vi "Main.vi"() -> ()   [LabVIEW 2013]
doc: "Use this template to build a simple state machine design pattern. Each state executes code and determines which state to transition to."
uses:
  <vilib>/express/express shared/transition.llb/Dynamic To Waveform Array.vi
  <vilib>/express/express shared/transition.llb/Waveform Array To Dynamic.vi
  <vilib>/express/express arith-compare/Formula/Block/exnFormulaBlock how many pts in the wave.vi
  <vilib>/express/express shared/ex_Modify Signal Name.vi
  <vilib>/express/express arith-compare/Formula/XNode/ExpressFormulaBlockNode.xnode
panel:
  out "Pwm Chart":i16(graph)
  out "PWM On":bool
  out "Mass Flow":dbl
  out "Bare, Coated, and DC":T1(graph)
  out "RecCount":i32
  in  "Period (ms)":dbl=3.0
  out "Coated Temperature":dbl
  out "Bare Temperature":dbl
  out "Low Airflow":bool
  in  "Stop":bool=TRUE
  in  "Filename to save to":path=path "Z:/adit/Desktop/MEL III/RefrigerationData.lvm" caption="Filename"
  in  "Save Data?":bool=TRUE
  out "Derivative Output":dbl
  out "Integral Output":dbl
  out "CO Bias":dbl
  out "Proportional Output":dbl
  out "Duty Cycle":dbl
  out "Current Set Point":dbl
  in  "Integral Constant":dbl=0.1 caption="I Coefficient" format="%0.2f"
  in  "Derivative \nConstant":dbl=0.05 caption="D Coefficient" format="%0.2f"
  in  "Proportional\nConstant":dbl=1.0 caption="P Coefficient" format="%0.2f"
  in  "Duty Cycle\nincrement amount":dbl=1.0
  in  "Decrease Duty Cycle":bool
  in  "Increase Duty Cycle":bool
  in  "Set Point\nIncrement amount":dbl=1.0
  in  "Lower Set Point":bool
  in  "Raise Set Point":bool
  in  "Bare(T) or \nCoated?":bool
  in  "Manual / Auto":bool
  in  "Time to wait(ms)":u32
  in  "Readings between\nrecorded data":i32
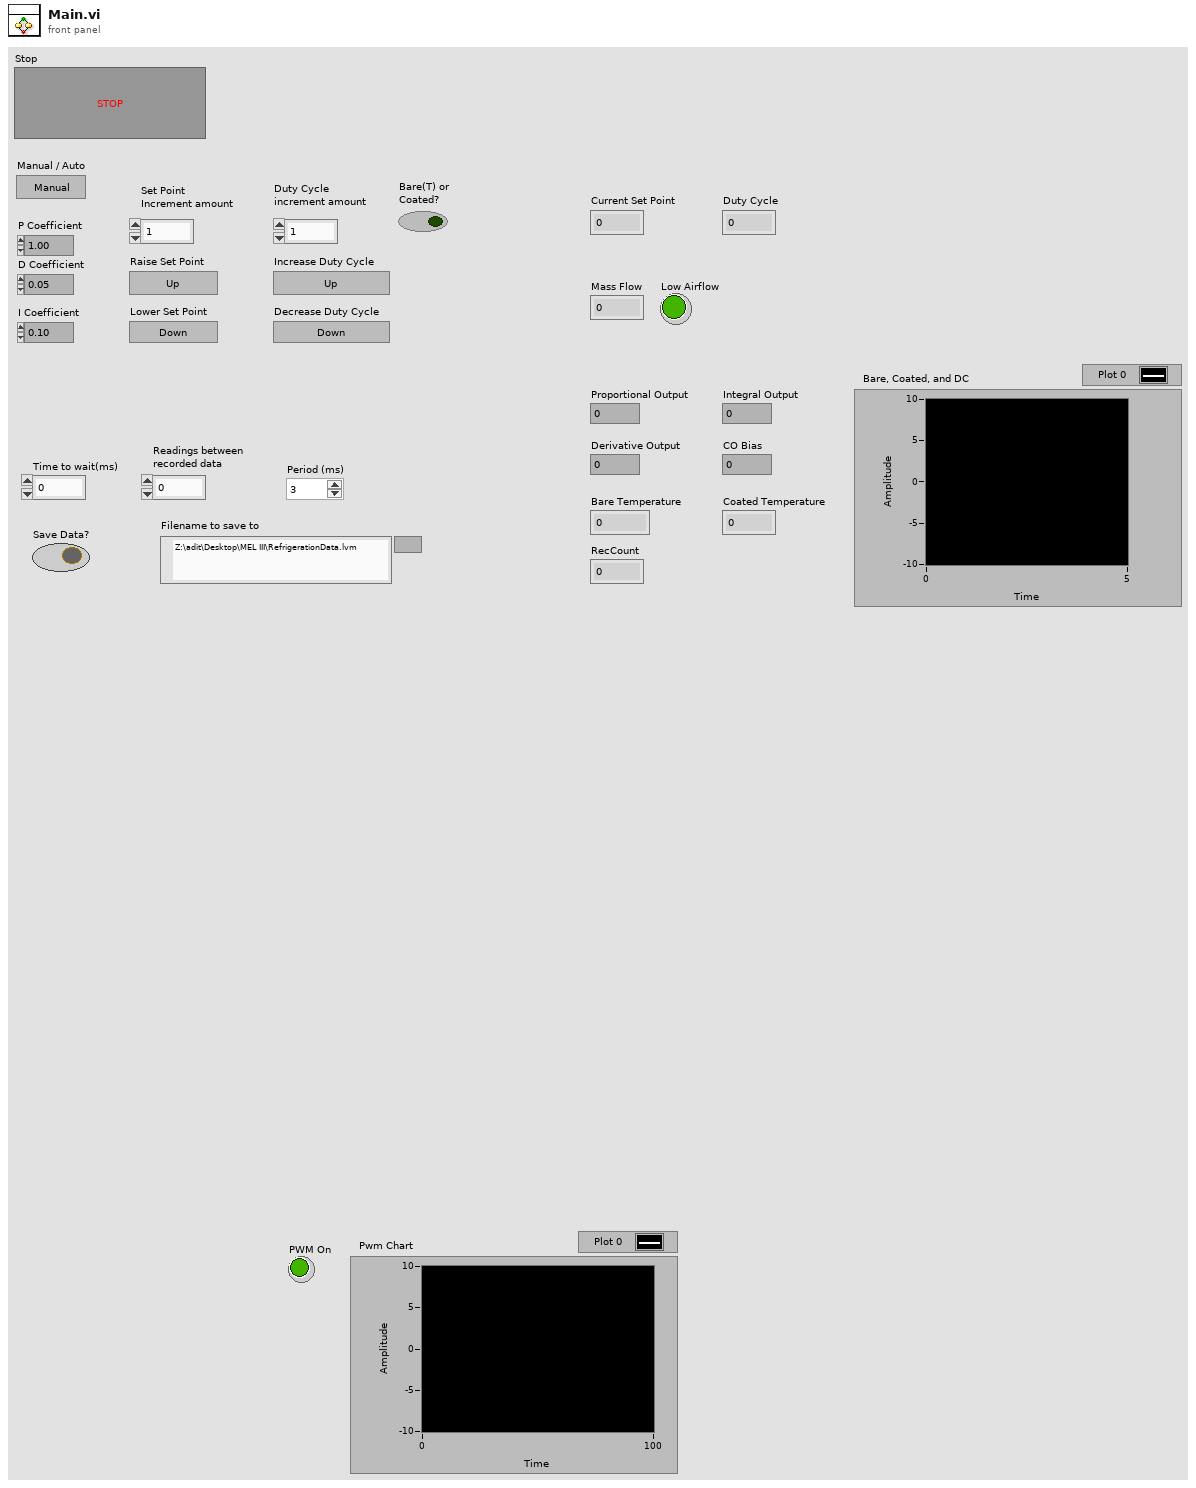
[diagram p1: front panel]
types:
  T1 = cluster{"Uncoated Probe":dbl, "Coated Probe":dbl, "Duty Cycle":dbl}
  T2 = cluster{"RecCount":i32, "Starting Tick Count":i32, "Coated Probe":dbl, "Uncoated Probe":dbl, "Mass Flow":dbl, "Derivative Out":dbl, "Integral Out":dbl, "Proportional Out":dbl, "Manual/Auto":bool, "Set Point":dbl, "Duty Cycle":dbl, "Pwm Value":bool}
  T3 = enum16{"Initialize", "Acquire", "Analyze", "PID", "Record", "PWM", "Output", ""}
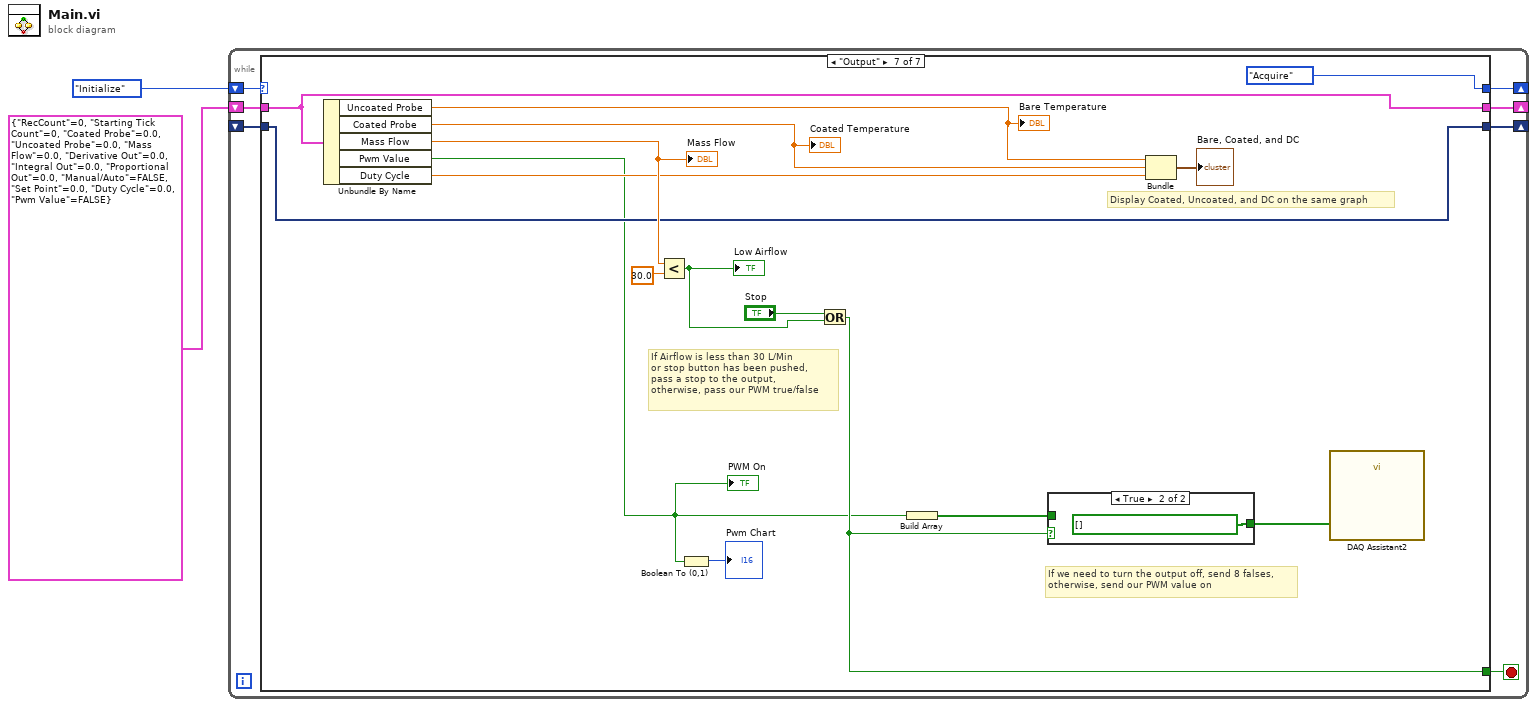
[diagram p0: block diagram]
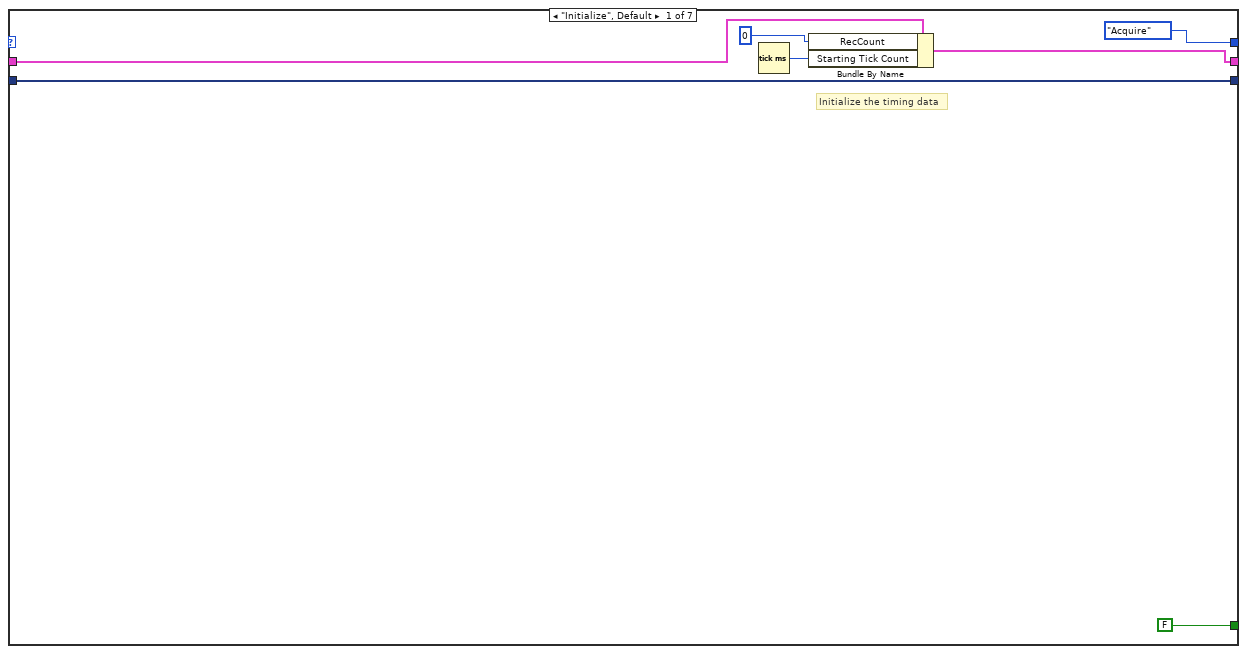
[diagram p2: hidden frame]
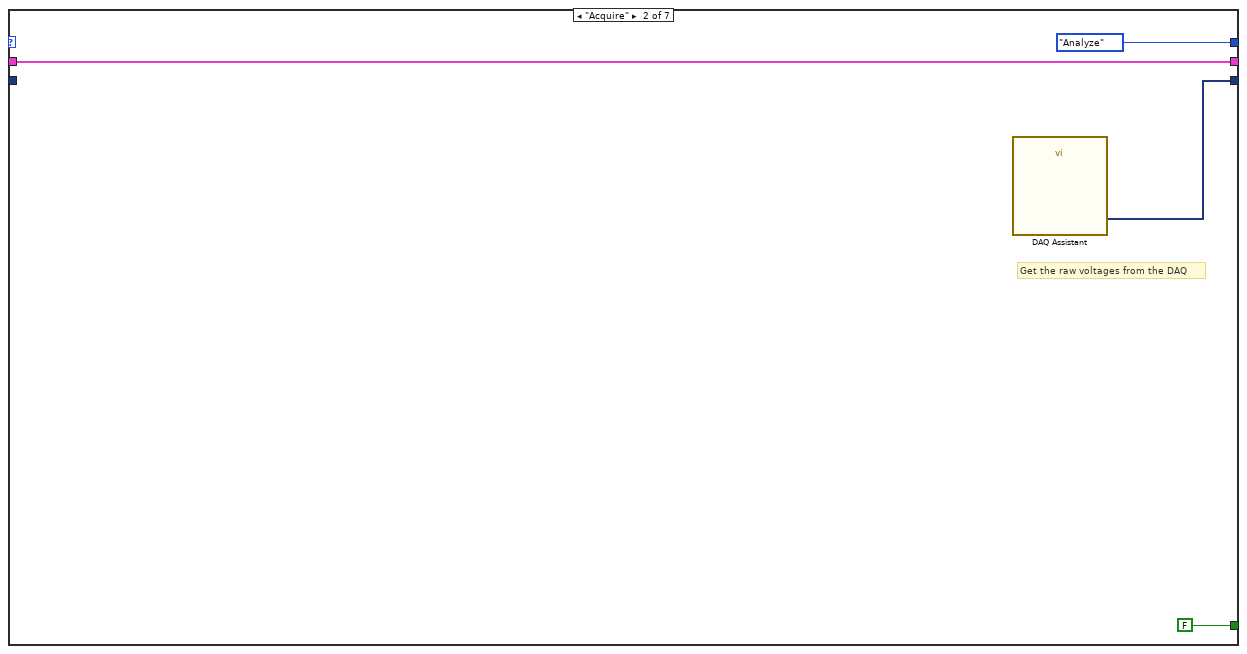
[diagram p3: hidden frame]
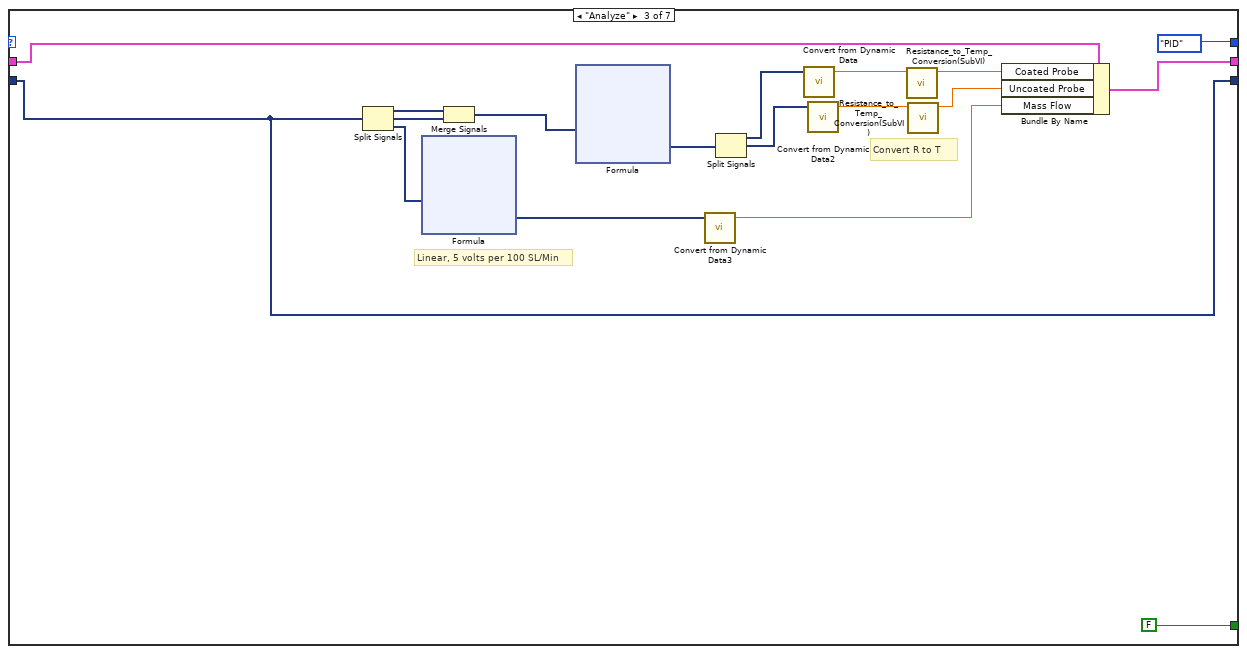
[diagram p4: hidden frame]
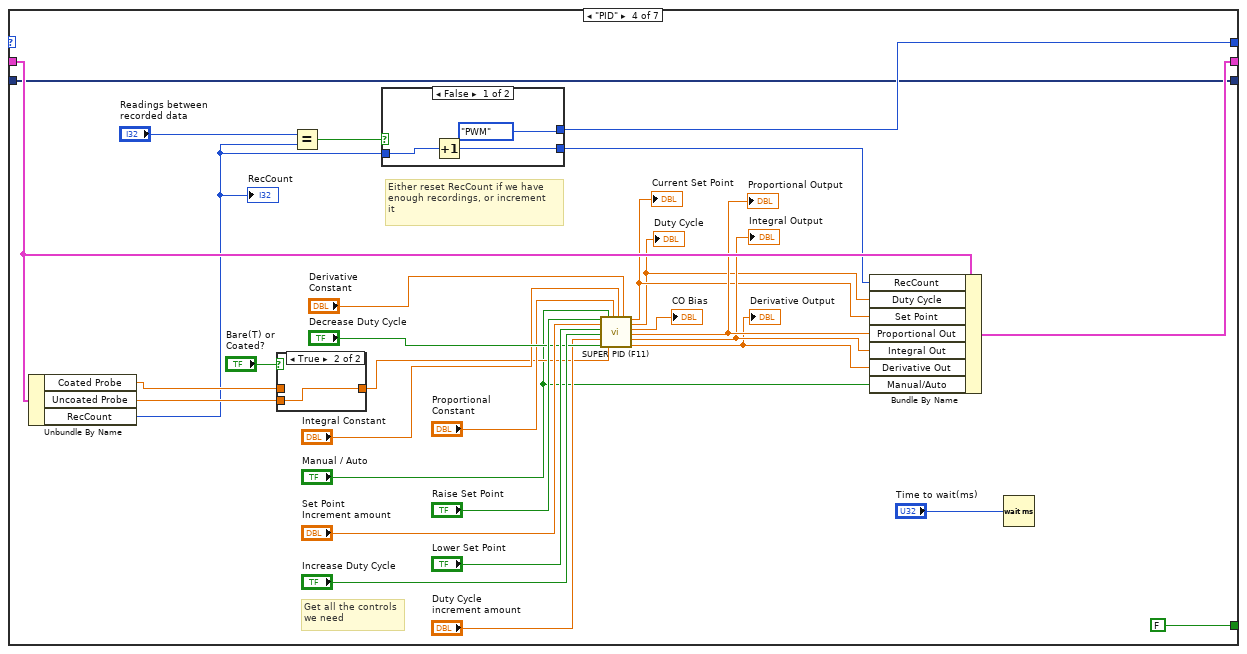
[diagram p5: hidden frame]
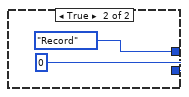
[diagram p7: hidden frame]
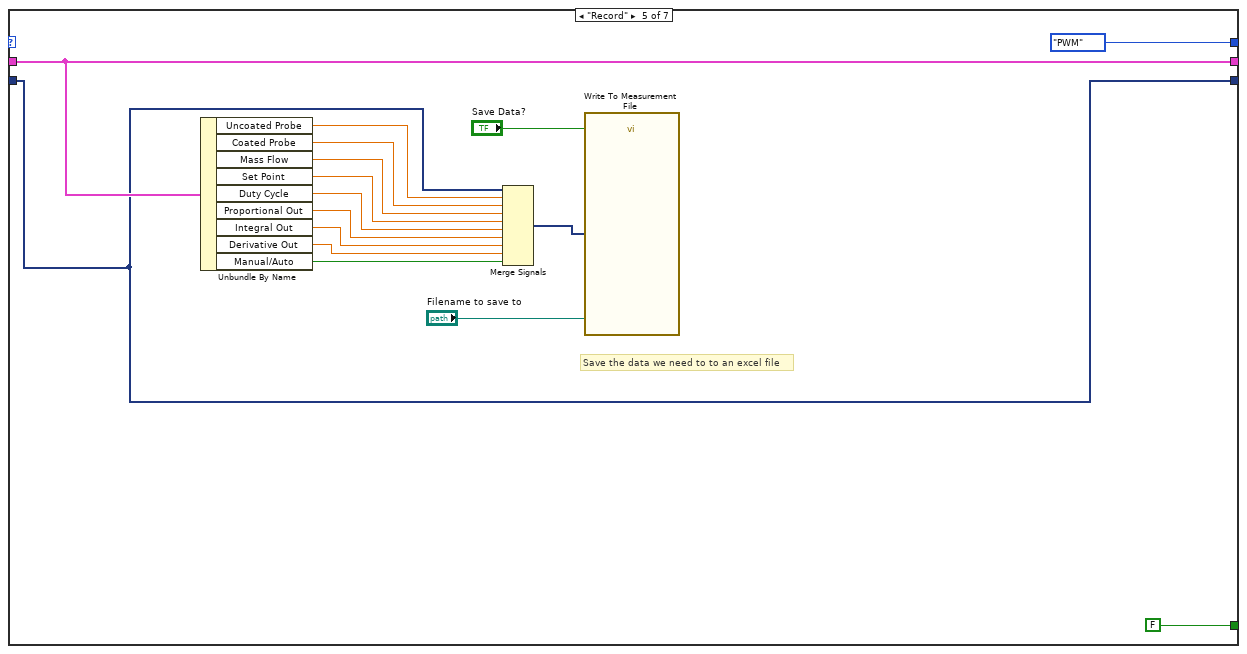
[diagram p8: hidden frame]
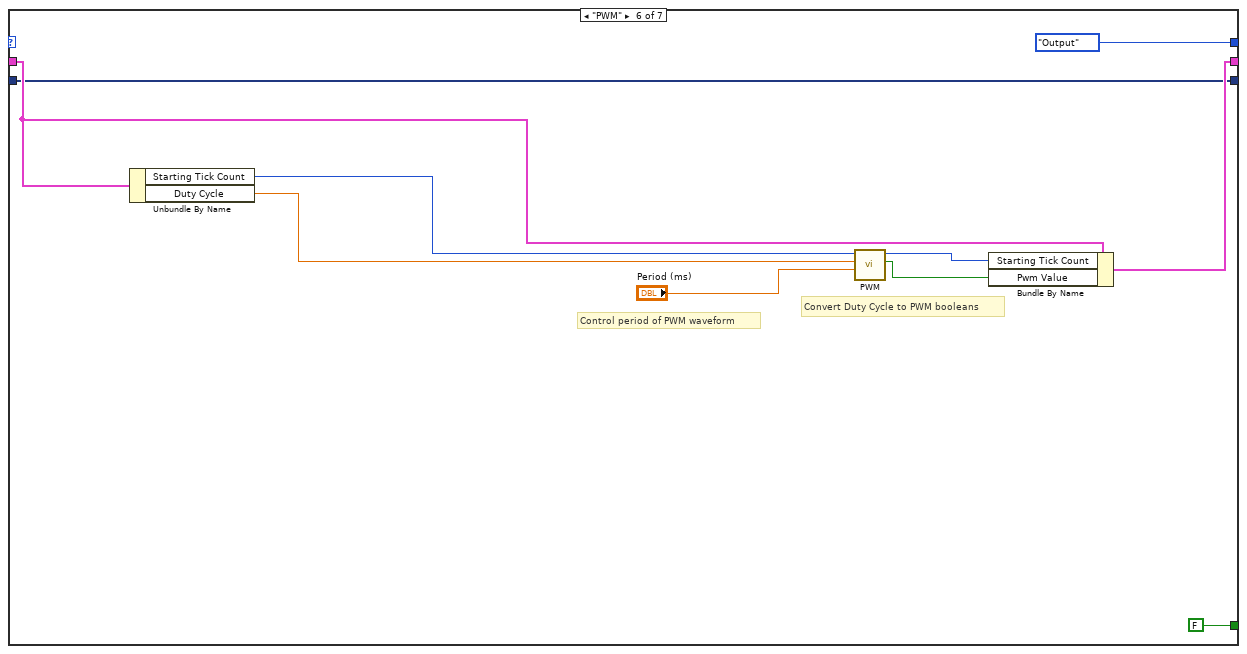
[diagram p9: hidden frame]
diagram:
  n1 = while {
    shift-right: [w8] -> _
    shift-left: T3."Initialize" -> [w9]
    shift-right: [w5] -> _
    shift-left: T2 {"RecCount"=0, "Starting Tick Count"=0, "Coated Probe"=0.0, "Uncoated Probe"=0.0, "Mass Flow"=0.0, "Derivative Out"=0.0, "Integral Out"=0.0, "Proportional Out"=0.0, "Manual/Auto"=FALSE, "Set Point"=0.0, "Duty Cycle"=0.0, "Pwm Value"=FALSE} -> [w6]
    shift-right: [w4] -> _
    shift-left: _ -> [w3]
    stop <- w7 stop-if-true
    n2 = case shown="\"Output\"" w9 {
      tunnel: [T3."Acquire" T3."Analyze" T3."PID" w334 T3."PWM" T3."Output" T3."Acquire"] -> w8
      tunnel: [FALSE FALSE FALSE ("Stop Loop?") FALSE ("Stop Loop?") FALSE FALSE w392] -> w7
      tunnel: [w13 w18 w24 w324 w354 w374 w390] -> w4
      tunnel: w6 -> [w16 w17 w28 w329 w356 w376 w389]
      tunnel: [w12 w17 w23 w325 w356 w375 w389] -> w5
      tunnel: w3 -> [w13 _ w24 w324 w354 w374 w390]
      frame "Initialize", Default {
        # "Initialize the timing data"
        n3 = Tick Count (ms)() -> (millisecond timer value=w14:u32)
        n4 = Bundle By Name(cluster=w16, "RecCount"=0, "Starting Tick Count"=w14) -> (w12:T2)
      }
      frame "Acquire" {
        # "Get the raw voltages from the DAQ"
        n5 = call "DAQ Assistant"() -> ("data"=w18:dynamicdata)  [unwired: 17 in, 2 out]
      }
      frame "Analyze" {
        # "Linear, 5 volts per 100 SL/Min"
        # "Convert R to T"
        n6 = Split Signals(w24) -> (w31:dynamicdata, w29:dynamicdata, w30:dynamicdata)  [unwired: 3 in]
        n7 = xnode "Formula"("V"=w30) -> ("Result"=w22:dynamicdata)  [unwired: 1 in, 1 out]
        n8 = Merge Signals(w31, w29) -> (w32:dynamicdata)
        n9 = xnode "Formula"("V"=w32) -> ("Result"=w37:dynamicdata)  [unwired: 1 in, 1 out]
        n10 = call "Convert from Dynamic Data3"("Dynamic Data Type"=w22) -> ("Scalar"=w21:dbl)  [unwired: 3 in]
        n11 = Split Signals(w37) -> (w36:dynamicdata, w35:dynamicdata)  [unwired: 3 in, 1 out]
        n12 = call "Convert from Dynamic Data"("Dynamic Data Type"=w36) -> ("Scalar"=w33:dbl)  [unwired: 3 in]
        n13 = call "Convert from Dynamic Data2"("Dynamic Data Type"=w35) -> ("Scalar"=w34:dbl)  [unwired: 3 in]
        n14 = call "Resistance_to_Temp_Conversion(SubVI).vi"("Scalar"=w33) -> ("Result"=w27:dbl)  [unwired: 10 in]
        n15 = call "Resistance_to_Temp_Conversion(SubVI).vi"("Scalar"=w34) -> ("Result"=w26:dbl)  [unwired: 10 in]
        n16 = Bundle By Name(cluster=w28, "Coated Probe"=w27, "Uncoated Probe"=w26, "Mass Flow"=w21) -> (w23:T2)
      }
      frame "PID" {
        # "Either reset RecCount if we have\nenough recordings, or increment\nit"
        # "Get all the controls\nwe need"
        n17 = Unbundle By Name(w329) -> ("Coated Probe"=w327:dbl, "Uncoated Probe"=w330:dbl, "RecCount"=w326:i32)
        "RecCount" <- w326
        n18 = case shown="True" "Bare(T) or \nCoated?" {
          tunnel: w327 -> [w347 _]
          tunnel: w330 -> [_ w348]
          tunnel: [w347 w348] -> w331
          frame False {
          }
          frame True {
          }
        }
        n19 = Equal?(x="Readings between\nrecorded data", y=w326) -> (x = y?=w336:bool)
        n20 = case shown="False" w336 {
          tunnel: [T3."PWM" T3."Record"] -> w334
          tunnel: [w350 0] -> w328
          tunnel: w326 -> [w349 _]
          frame False {
            n21 = Increment(x=w349) -> (x+1=w350:i32)
          }
          frame True {
          }
        }
        n22 = call "SUPER PID (F11).vi"("SP Up"="Raise Set Point", "SP Increment"="Set Point\nIncrement amount", "SP Down"="Lower Set Point", "DC Up"="Increase Duty Cycle", "DC Increment"="Duty Cycle\nincrement amount", "DC Down"="Decrease Duty Cycle", "Manual / Auto"="Manual / Auto", "PV"=w331, "P"="Proportional\nConstant", "I"="Integral Constant", "D"="Derivative \nConstant") -> ("SP"=w319:dbl, "DC"=w318:dbl, "CO Bias"=→"CO Bias":dbl, "P out"=w323:dbl, "I out"=w322:dbl, "D out"=w321:dbl)  [unwired: 3 in]
        "Current Set Point" <- w319
        "Duty Cycle" <- w318
        "Proportional Output" <- w323
        "Integral Output" <- w322
        "Derivative Output" <- w321
        n23 = Bundle By Name(cluster=w329, "RecCount"=w328, "Duty Cycle"=w318, "Set Point"=w319, "Proportional Out"=w323, "Integral Out"=w322, "Derivative Out"=w321, "Manual/Auto"="Manual / Auto") -> (w325:T2)
        n24 = Wait (ms)(milliseconds to wait="Time to wait(ms)") -> ()  [unwired: 1 out]
      }
      frame "Record" {
        # "Save the data we need to to an excel file"
        n25 = Unbundle By Name(w356) -> ("Uncoated Probe"=w355:dbl, "Coated Probe"=w366:dbl, "Mass Flow"=w365:dbl, "Set Point"=w358:dbl, "Duty Cycle"=w364:dbl, "Proportional Out"=w363:dbl, "Integral Out"=w357:dbl, "Derivative Out"=w360:dbl, "Manual/Auto"=w359:bool)
        n26 = Merge Signals(w354, w355, w366, w365, w358, w364, w363, w357, w360, w359) -> (w367:dynamicdata)
        n27 = call "Write To Measurement File"("Signals"=w367, "Reset"="Save Data?", "Filename"="Filename to save to") -> ()  [unwired: 14 in, 3 out]
      }
      frame "PWM" {
        # "Control period of PWM waveform"
        # "Convert Duty Cycle to PWM booleans"
        n28 = Unbundle By Name(w376) -> ("Starting Tick Count"=w372:i32, "Duty Cycle"=w377:dbl)
        n29 = call "PWM.vi"("Period (ms)"="Period (ms)", "Duty Cycle"=w377, "Starting Tick Count"=w372) -> ("Pwm value"=w370:bool, "Starting Tick Count"=w371:u32)  [unwired: 7 in]
        n30 = Bundle By Name(cluster=w376, "Starting Tick Count"=w371, "Pwm Value"=w370) -> (w375:T2)
      }
      frame "Output" {
        # "If we need to turn the output off, send 8 falses, \notherwise, send our PWM value on"
        # "Display Coated, Uncoated, and DC on the same graph"
        # "If Airflow is less than 30 L/Min\nor stop button has been pushed, \npass a stop to the output,\notherwise, pass our PWM true/false"
        n31 = Unbundle By Name(w389) -> ("Uncoated Probe"=w387:dbl, "Coated Probe"=w386:dbl, "Mass Flow"=w393:dbl, "Pwm Value"=w380:bool, "Duty Cycle"=w385:dbl)
        "Bare Temperature" <- w387
        "Coated Temperature" <- w386
        "Mass Flow" <- w393
        "PWM On" <- w380
        n32 = Less?(x=w393, y=30.0) -> (x < y?=w383:bool)
        "Low Airflow" <- w383
        n33 = Boolean To (0,1)(Boolean=w380) -> (0, 1=→"Pwm Chart":i16)
        n34 = Or(x="Stop", y=w383) -> (x .or. y?=w392:bool)
        n35 = Build Array(w380) -> (w391:bool[])
        n36 = case shown="True" w392 {
          tunnel: [w396 bool[] []] -> w384
          tunnel: w391 -> [w396 _]
          frame False {
          }
          frame True {
          }
        }
        n37 = Bundle("Uncoated Probe"=w387, "Coated Probe"=w386, "Duty Cycle"=w385) -> (→"Bare, Coated, and DC":T1)  [unwired: 1 in]
        n38 = call "DAQ Assistant2"("data"=w384) -> ()  [unwired: 17 in, 2 out]
      }
    }
  }
